vi "Periodic Tasks.vi"(8 "error in":errorcluster) -> ()   [LabVIEW 2014]
doc: "This VI runs in parallel to other tasks. It can contain as many user-defined periodic loops as you need. These can carry out PID or other sorts of timed response."
uses:
  <vilib>/Rock Robotics/WPI/DriverStation/WPI_DriverStationRobotMode2.ctl
  <vilib>/Rock Robotics/WPI/Solenoid/WPI_SolenoidValue.ctl
  <vilib>/Rock Robotics/WPI/RobotDrive/WPI_RobotDriveGetSetRefNum.vi
  <vilib>/Rock Robotics/WPI/Joystick/WPI_JoystickGetSetRefNum.vi
  <vilib>/Rock Robotics/Network Tables/SD Read Boolean.vi
  Robot Global Data.vi
  <vilib>/Rock Robotics/Network Tables/SD Write Boolean.vi
  <vilib>/addons/control/pid/pid.llb/PID (DBL).vi
  <vilib>/Rock Robotics/Network Tables/SD Write Number.vi
  <vilib>/Rock Robotics/WPI/Compressor/WPI_CompressorGetSetRefNum.vi
  Moose Code/Auto_Conf.vi
  <vilib>/Rock Robotics/WPI/Solenoid/WPI_SolenoidSetEnum.vi
  <vilib>/Rock Robotics/WPI/Solenoid/Deprecated/WPI_SolenoidSetBool.vi
  <vilib>/addons/control/pid/NI_PID_pid.lvlib
panel:
  out "Boolean":bool
  in  "Kpd":dbl=0.015
  in  "AllowZero":bool
  in  "ElevatorReset":bool
  out "GoatDetectorPhotoeye":bool
  out "D Contribution":dbl
  in  "Kd":dbl=0.025
  out "BottomOvertravel":bool=TRUE
  out "TopOvertravel":bool=TRUE
  out "ElevatorCurrent":dbl
  out "Voltage":dbl
  out "CurrentSum":dbl
  out "Motor Control":dbl(graph)
  in  "IZone":dbl=20.0
  out "Current":dbl
  out "Target":dbl
  out "PIDPhotoeye":bool
  in  "Kp":dbl=0.027
  in  "Ki":dbl=0.002 step=0.0001
  out "Target vs. Actual":T1(graph)
  out "I Contribution":dbl
  out "P Contribution":dbl
  in  "Threshold":dbl=5.5
  out "In Position":bool
  out "EncoderLeft":dbl
  out "EncoderRight":dbl
  # "K's as of 4-16-2015\nKp=0.027\nKpd=0.015\nKi=0.002\nKd=0.025\nIZone=20\nThreshold=5.5"
  # "K Tune-torial: (copied from Mindstorms docs)\n      Set the values of Ki, Kd"
  # "K Tune-torial: (copied from email)\n      Find a P gain that gets you close to your target without overshooting.  \nBased on that P gain value calculate the error at which your P starts to\ndecrease below full throttle.  Make your I cap equal to this error.  Make your\ninitial I gain very small (less than .1 say .0001).  The idea is to accumulate a \nvalue that is manageable. The Talon I accumulates every 1 millisecond so it\nis very easy to calculate the amount of time to get to full throttle.  An I gain\nof .001 will get you full throttle in about 1 second (assuming error never\nchanges).\n      The goal of this strategy is to make I perceivable while still allowing\nP to be the dominating component.  In position servo, I is only needed\nwhen P is not enough to get you to your target.  Once your P output is\nless than full throttle, I will start to kick in.  At first there will be a noticeable\ngap in throttle.  Throttle will decrease proportional to the error and then\nslowly ramp back up until the target is reached, this is useful in observing\nthe effect of I.  Slowly increase I and adjust the I zone until the throttle is \nalmost seamless."
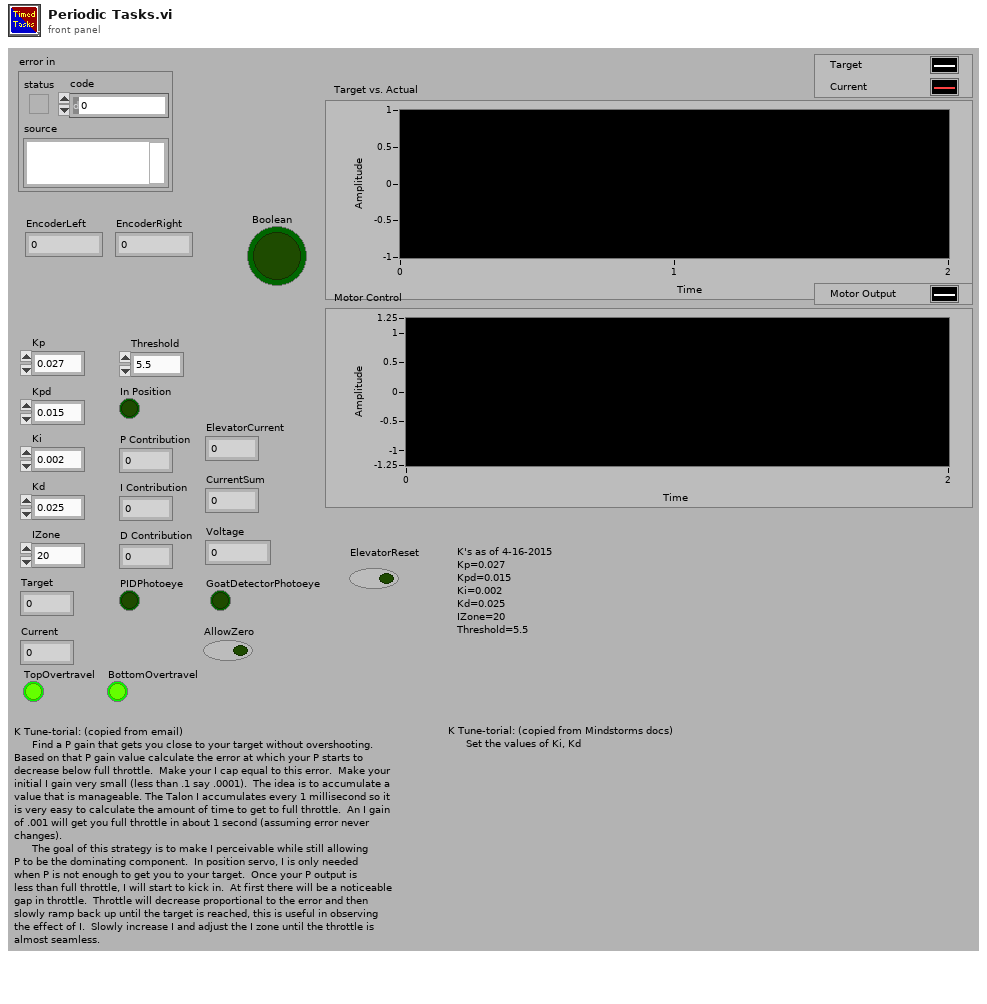
[diagram p1: front panel]
types:
  T1 = cluster{"[0]":dbl, "[1]":dbl, "[2]":dbl, "[3]":dbl, "[4]":dbl, "[5]":dbl, "[6]":dbl, "[7]":dbl, "[8]":dbl}
  T2 = enum16{"ResetForward", "ResetBack", "PIDControl", "ManualControl", "ZeroEncoderAndTarget", "AutoStack"}
  T3 = enum16{"Disabled", "Initialize", "CalcNewTarget", "Moving", "OpenArm", "CloseArm", "Reset"}
  T4 = typedef "WPI_EncoderDevRef.ctl" = cluster{"DevStatus":errorcluster, "EncoderIndex":T5, "CounterIndex":T6, "DistancePerCount":dbl, "Decoding Type":T7}
  T5 = typedef "FPGA_EncoderIdx.ctl" = enum8{"Enc 0", "Enc 1", "Enc 2", "Enc 3", "Enc 4", "Enc 5", "Enc 6", "Enc 7", "Invalid"}
  T6 = typedef "FPGA_CounterCtrSystemIndex.ctl" = enum8{"Ctr 0", "Ctr 1", "Ctr 2", "Ctr 3", "Ctr 4", "Ctr 5", "Ctr 6", "Ctr 7", "Invalid"}
  T7 = typedef "WPI_EncoderType.ctl" = enum16{"1x", "2x", "4x"}
  T8 = typedef "WPI_JoystickDevRef.ctl" = cluster{"Device":T9}
  T9 = typedef "WPI_JoystickDeviceEnum.ctl" = enum16{"USB 0", "USB 1", "USB 2", "USB 3", "USB 4", "USB 5"}
  T10 = typedef "WPI_SolenoidDevRef.ctl" = cluster{"DevStatus":errorcluster, "Pneumatics Control Module":u8, "Forward Solenoid Channel":T11, "Reverse Solenoid Channel":T11}
  T11 = typedef "WPI_SolenoidChannel.ctl" = enum8{"Solenoid 0", "Solenoid 1", "Solenoid 2", "Solenoid 3", "Solenoid 4", "Solenoid 5", "Solenoid 6", "Solenoid 7", "Invalid"}
  T12 = typedef "WPI_MotorControlDeviceRef.ctl" = cluster{"DeviceStatus":errorcluster, "Type":T13, "PWM":cluster{"Controller":T14, "PWM Channel":T15, "DeadBand":T16}, "CAN":cluster{"Device Number":u8, "Control Mode":T17, "Semaphore":T18, "Max Vout":dbl, "TalonSRX Control Mode":T19}, "Invert":bool, "TransformRef":T20, "InvTransformRef":T20}
  T13 = typedef "WPI_MotorControlType.ctl" = enum16{"PWM", "CAN", "CANTalonSRX"}
  T14 = typedef "FPGA_TypedefDigitalModule.ctl" = enum16{"Controller 1"}
  T15 = typedef "FPGA_DIOPWMChannel.ctl" = enum8{"PWM 0", "PWM 1", "PWM 2", "PWM 3", "PWM 4", "PWM 5", "PWM 6", "PWM 7", "PWM 8", "PWM 9", "PWM MXP 0", "PWM MXP 1", "PWM MXP 2", "PWM MXP 3", "PWM MXP 4", "PWM MXP 5", "PWM MXP 6", "PWM MXP 7", "PWM MXP 8", "PWM MXP 9", "Invalid"}
  T16 = typedef "WPI_PWMDeadband.ctl" = cluster{"Name":string, "maxPositivePwm":i32, "minPositivePwm":i32, "centerPwm":i32, "maxNegativePwm":i32, "minNegativePwm":i32, "angularRange":u16}
  T17 = typedef "WPI_CANJaguar_ControlMode.ctl" = enum8{"Percent VBus", "Current", "Speed", "Position", "Voltage"}
  T18 = typedef "Semaphore RefNum" = refnum<k1>
  T19 = typedef "WPI_CANTalonSRX_APIControlMode.ctl" = enum8{"Percent VBus", "Speed", "Position", "Slave", "Unchanged / Invalid"}
  T20 = typedef "WPI_PWMTransform_ConPane.ctl" = refnum<vi>
  T21 = typedef "WPI_RobotDriveDevRef.ctl" = cluster{"DevStatus":errorcluster, "Motors[]":T12[], "Square Inputs":bool, "Max Output":dbl}
  T22 = typedef "WPI_DigitalInputDevRef.ctl" = cluster{"DevStatus":errorcluster, "DIO Channel":T23, "Controller":T14}
  T23 = typedef "FPGA_DIOChannel.ctl" = enum8{"DIO 0", "DIO 1", "DIO 2", "DIO 3", "DIO 4", "DIO 5", "DIO 6", "DIO 7", "DIO 8", "DIO 9", "DIO MXP 0", "DIO MXP 1", "DIO MXP 2", "DIO MXP 3", "DIO MXP 4", "DIO MXP 5", "DIO MXP 6", "DIO MXP 7", "DIO MXP 8", "DIO MXP 9", "DIO MXP 10", "DIO MXP 11", "DIO MXP 12", "DIO MXP 13", "DIO MXP 14", "DIO MXP 15", "Invalid"}
  T24 = typedef "WPI_CompressorDevRef.ctl" = cluster{"DevStatus":errorcluster, "Pneumatics Control Module":u8}
  T25 = typedef "WPI_DriverStationRobotMode2.ctl" = enum16{"Autonomous Disabled", "Autonomous Enabled", "Teleop Disabled", "Teleop Enabled", "Disconnected", "Finish", "Test Disabled", "Test Enabled", "Emergency Stopped"}
  T26 = typedef "WPI_GyroDevRef.ctl" = cluster{"DevStatus":errorcluster, "Analog Module":T27, "Analog Channel":T28, "Offset":dbl, "Gain (VoltsPerDegree/Second)":dbl}
  T27 = typedef "FPGA_TypedefAnalogModule.ctl" = enum16{"Controller 1"}
  T28 = typedef "FPGA_AIChannel.ctl" = enum8{"AI 0", "AI 1", "AI 2", "AI 3", "AI MXP 0", "AI MXP 1", "AI MXP 2", "AI MXP 3", "Invalid"}
  T29 = typedef "WPI_SolenoidValue.ctl" = enum16{"Off", "On", "Forward", "Reverse"}
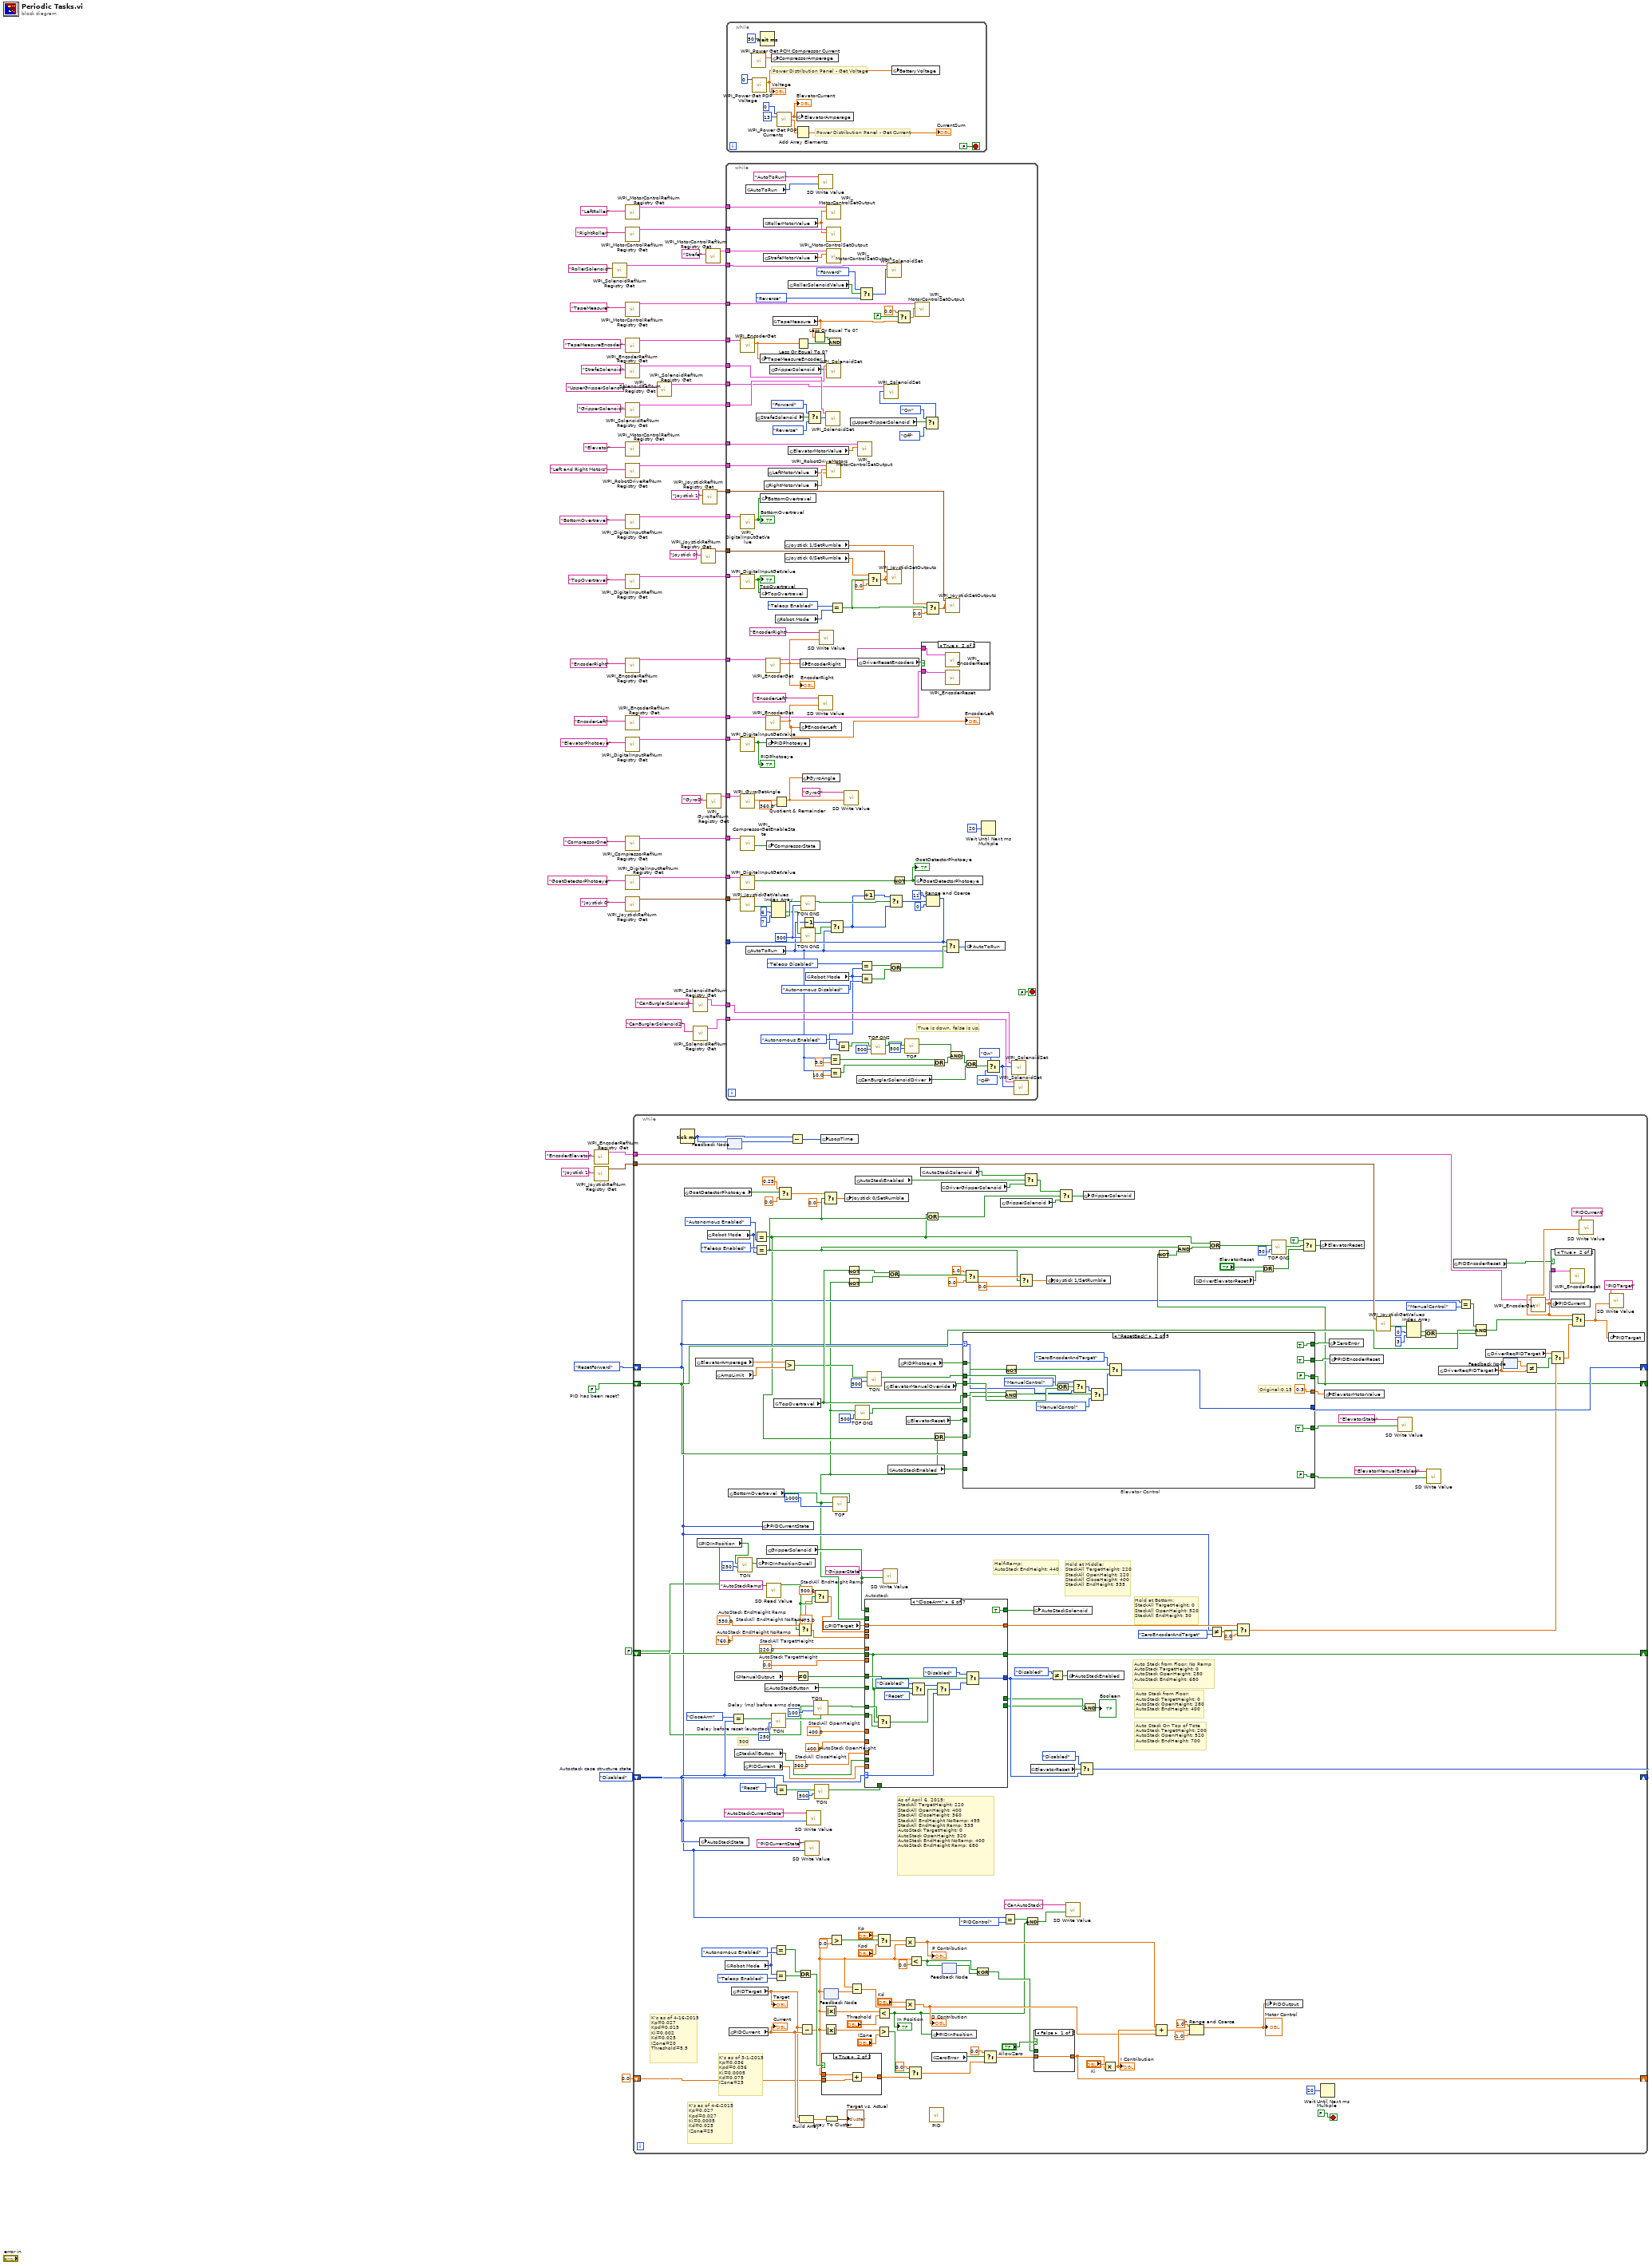
[diagram p0: block diagram]
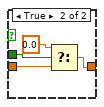
[diagram p4: hidden frame]
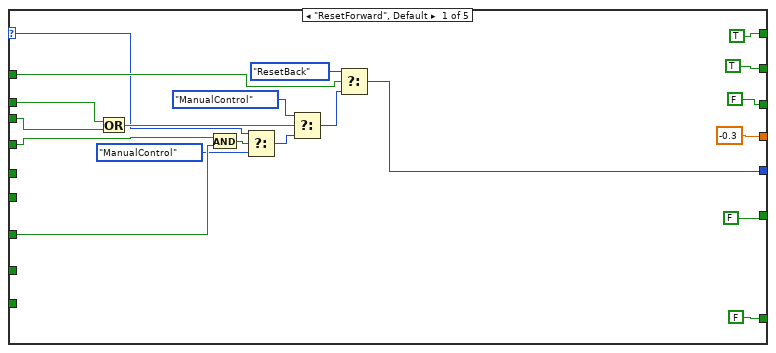
[diagram p5: hidden frame]
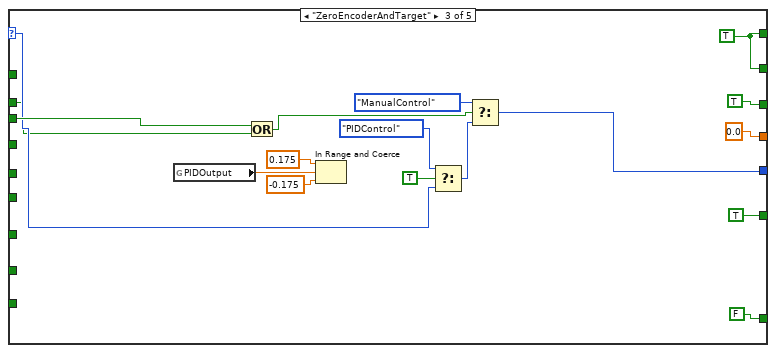
[diagram p6: hidden frame]
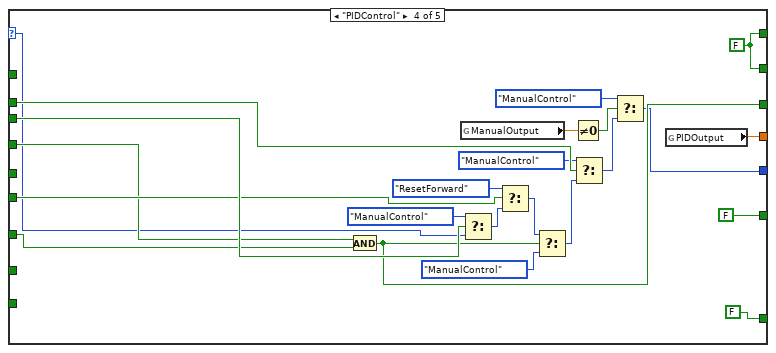
[diagram p7: hidden frame]
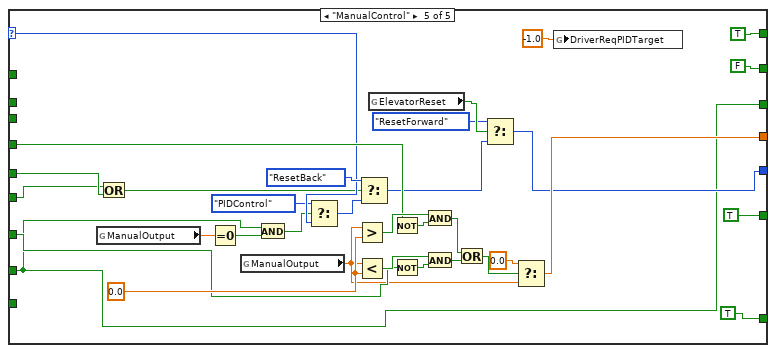
[diagram p8: hidden frame]
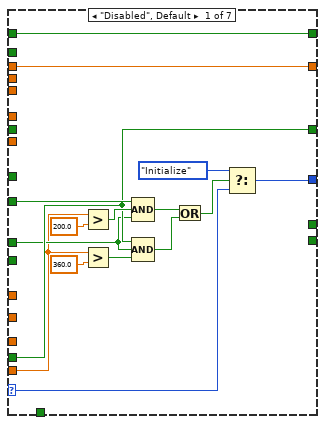
[diagram p9: hidden frame]
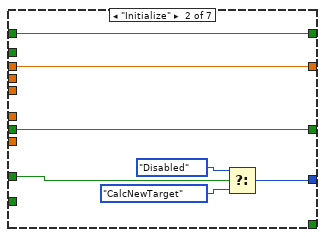
[diagram p10: hidden frame]
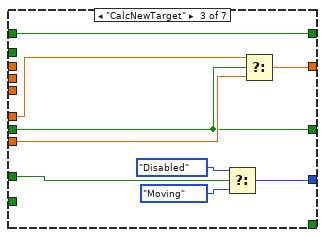
[diagram p11: hidden frame]
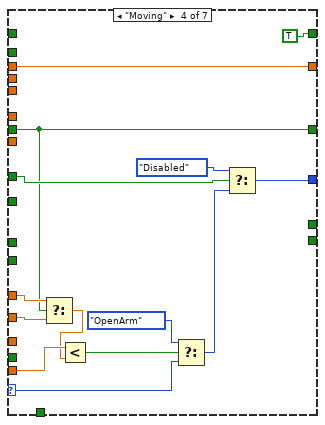
[diagram p12: hidden frame]
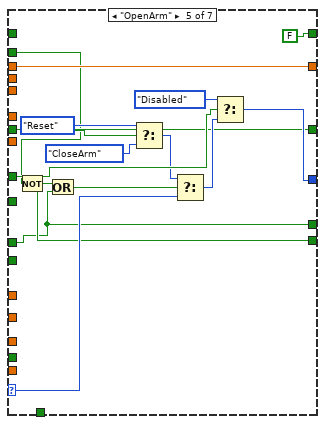
[diagram p13: hidden frame]
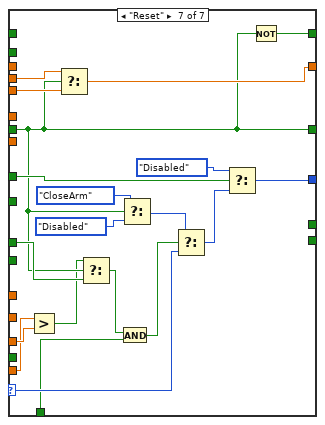
[diagram p14: hidden frame]
diagram:
  w28 = FALSE  # PID has been reset?
  w31 = T3."Disabled"  # Autostack case structure state
  n1 = call <vilib>:"WPI_EncoderRefNum Registry Get.vi"("refnum name"="EncoderElevator") -> ("EncoderDevRef"=w17:T4)  [unwired: 9 in, 1 out]
  n2 = call <vilib>:"WPI_JoystickRefNum Registry Get.vi"("refnum name"="Joystick 1") -> ("JoystickDevRef"=w15:T8)  [unwired: 9 in, 1 out]
  n3 = call <vilib>:"WPI_SolenoidRefNum Registry Get.vi"("refnum name"="RollerSolenoid") -> ("SolenoidDevRef"=w18:T10)  [unwired: 9 in, 1 out]
  n4 = call <vilib>:"WPI_MotorControlRefNum Registry Get.vi"("refnum name"="LeftRoller") -> ("MotorControlDevRef"=w21:T12)  [unwired: 9 in, 1 out]
  n5 = call <vilib>:"WPI_MotorControlRefNum Registry Get.vi"("refnum name"="RightRoller") -> ("MotorControlDevRef"=w20:T12)  [unwired: 9 in, 1 out]
  n6 = call <vilib>:"WPI_MotorControlRefNum Registry Get.vi"("refnum name"="TapeMeasure") -> ("MotorControlDevRef"=w12:T12)  [unwired: 9 in, 1 out]
  n7 = call <vilib>:"WPI_EncoderRefNum Registry Get.vi"("refnum name"="TapeMeasureEncoder") -> ("EncoderDevRef"=w9:T4)  [unwired: 9 in, 1 out]
  n8 = call <vilib>:"WPI_SolenoidRefNum Registry Get.vi"("refnum name"="StrafeSolenoid") -> ("SolenoidDevRef"=w24:T10)  [unwired: 9 in, 1 out]
  n9 = call <vilib>:"WPI_SolenoidRefNum Registry Get.vi"("refnum name"="GripperSolenoid") -> ("SolenoidDevRef"=w6:T10)  [unwired: 9 in, 1 out]
  n10 = call <vilib>:"WPI_MotorControlRefNum Registry Get.vi"("refnum name"="Elevator") -> ("MotorControlDevRef"=w5:T12)  [unwired: 9 in, 1 out]
  n11 = call <vilib>:"WPI_RobotDriveRefNum Registry Get.vi"("refnum name"="Left and Right Motors") -> ("RobotDriveDevRef"=w57:T21)  [unwired: 9 in, 1 out]
  n12 = call <vilib>:"WPI_DigitalInputRefNum Registry Get.vi"("refnum name"="BottomOvertravel") -> ("DigitalInputDevRef"=w39:T22)  [unwired: 9 in, 1 out]
  n13 = call <vilib>:"WPI_DigitalInputRefNum Registry Get.vi"("refnum name"="TopOvertravel") -> ("DigitalInputDevRef"=w41:T22)  [unwired: 9 in, 1 out]
  n14 = call <vilib>:"WPI_EncoderRefNum Registry Get.vi"("refnum name"="EncoderRight") -> ("EncoderDevRef"=w46:T4)  [unwired: 9 in, 1 out]
  n15 = call <vilib>:"WPI_EncoderRefNum Registry Get.vi"("refnum name"="EncoderLeft") -> ("EncoderDevRef"=w48:T4)  [unwired: 9 in, 1 out]
  n16 = call <vilib>:"WPI_DigitalInputRefNum Registry Get.vi"("refnum name"="ElevatorPhotoeye") -> ("DigitalInputDevRef"=w51:T22)  [unwired: 9 in, 1 out]
  n17 = call <vilib>:"WPI_CompressorRefNum Registry Get.vi"("refnum name"="CompressorOne") -> ("CompressorDevRef"=w13:T24)  [unwired: 9 in, 1 out]
  n18 = call <vilib>:"WPI_DigitalInputRefNum Registry Get.vi"("refnum name"="GoatDetectorPhotoeye") -> ("DigitalInputDevRef"=w32:T22)  [unwired: 9 in, 1 out]
  n19 = call <vilib>:"WPI_JoystickRefNum Registry Get.vi"("refnum name"="Joystick 0") -> ("JoystickDevRef"=w26:T8)  [unwired: 9 in, 1 out]
  n20 = while {
    shift-right: [w164] -> _
    shift-left: 0.0 -> [w103]
    shift-right: [w154] -> _
    shift-left: w31 -> [w85]
    shift-right: [w227] -> _
    shift-left: FALSE -> [w228]
    shift-right: [w189] -> _
    shift-left: T2."ResetForward" -> [w66]
    shift-right: [w97] -> _
    shift-left: w28 -> [w138]
    tunnel: w17 -> [w72]
    tunnel: w15 -> [w127]
    stop <- FALSE stop-if-true
    w68 = 475.0  # StackAll EndHeight NoRamp
    w70 = 500.0  # StackAll EndHeight Ramp
    w73 = 760.0  # AutoStack EndHeight NoRamp
    w82 = 360.0  # StackAll CloseHeight
    w91 = 400.0  # StackAll OpenHeight
    w90 = 400.0  # AutoStack OpenHeight
    w92 = 220.0  # StackAll TargetHeight
    w74 = 530.0  # AutoStack EndHeight Ramp
    w141 = 0.0  # AutoStack TargetHeight
    w148 = u32 250  # Delay before reset (autostack)
    w156 = u32 100  # Delay (ms) before arms close
    # "K's as of 4-16-2015\nKp=0.027\nKpd=0.015\nKi=0.002\nKd=0.025\nIZone=20\nThreshold=5.5"
    # "500"
    # "As of April 6, 2015:\nStackAll TargetHeight: 220\nStackAll OpenHeight: 400\nStackAll CloseHeight: 360\nStackAll EndHeight NoRamp: 495 \nStackAll EndHeight Ramp: 535\nAutoStack TargetHeight: 0\nAutoStack OpenHeight: 320\nAutoStack EndHeight NoRamp: 400\nAutoStack EndHeight Ramp: 680"
    # "K's as of 4-6-2015\nKp=0.027\nKpd=0.027\nKi=0.0005\nKd=0.025\nIZone=25"
    # "Auto Stack from Floor: No Ramp\nAutoStack TargetHeight: 0\nAutoStack OpenHeight: 280\nAutoStack EndHeight: 680"
    # "Half-Ramp:\nAutoStack EndHeight: 440"
    # "Hold at Bottom:\nStackAll TargetHeight: 0\nStackAll OpenHeight: 520\nStackAll EndHeight: 30"
    # "Auto Stack On Top of Tote\nAutoStack TargetHeight: 200\nAutoStack OpenHeight: 520\nAutoStack EndHeight: 700"
    # "Auto Stack from Floor:\nAutoStack TargetHeight: 0\nAutoStack OpenHeight: 280\nAutoStack EndHeight: 400"
    # "Hold at Middle:\nStackAll TargetHeight: 220\nStackAll OpenHeight: 220\nStackAll CloseHeight: 400\nStackAll EndHeight: 535"
    # "K's as of 3-1-2015\nKp=0.036\nKpd=0.036\nKi=0.0005\nKd=0.075\nIZone=25"
    n21 = Tick Count (ms)() -> (millisecond timer value=w173:u32)
    n22 = global read "Robot Global Data.vi" "GoatDetectorPhotoeye"() -> (w222:bool)
    n23 = global read "Robot Global Data.vi" "ElevatorAmperage"() -> (w200:dbl)
    n24 = global read "Robot Global Data.vi" "PIDInPosition"() -> (w63:bool)
    n25 = global write "Robot Global Data.vi" "AutoStackState"(w85) -> ()
    n26 = global read "Robot Global Data.vi" "Robot Mode"() -> (w98:T25)
    n27 = global read "Robot Global Data.vi" "AmpLimit"() -> (w201:dbl)
    n28 = global read "Robot Global Data.vi" "Robot Mode"() -> (w107:T25)
    n29 = feedback-in #1(w173) -> ()
    n30 = feedback #1() -> (w172:u32)  [unwired: 1 in]
    n31 = global read "Robot Global Data.vi" "BottomOvertravel"() -> (w62:bool)
    n32 = global read "Robot Global Data.vi" "PIDCurrent"() -> (w241:dbl)
    "Current" <- w241
    n33 = Equal?(x=T3."CloseArm" ("t"), y=w85) -> (x = y?=w149:bool)
    n34 = global read "Robot Global Data.vi" "PIDTarget"() -> (w237:dbl)
    "Target" <- w237
    n35 = global read "Robot Global Data.vi" "ManualOutput"() -> (w140:dbl)
    n36 = global read "Robot Global Data.vi" "StackAllButton"() -> (w83:bool)
    n37 = call "TON.vi"("Delay (ms)"=u32 250, "Input"=w63) -> ("Output"=w134:bool)  [unwired: 9 in]
    n38 = global read "Robot Global Data.vi" "PIDCurrent"() -> (w84:dbl)
    n39 = Equal?(x=w98, y=WPI_DriverStationRobotMode2."Autonomous Enabled") -> (x = y?=w113:bool)
    n40 = Equal?(x=WPI_DriverStationRobotMode2."Teleop Enabled" ("y"), y=w98) -> (x = y?=w115:bool)
    n41 = global write "Robot Global Data.vi" "PIDInPositionDwell"(w134) -> ()
    n42 = global write "Robot Global Data.vi" "PIDCurrentState"(w66) -> ()
    n43 = global read "Robot Global Data.vi" "AutoStackButton"() -> (w67:bool)
    n44 = global read "Robot Global Data.vi" "GripperSolenoid"() -> (w123:bool)
    n45 = call-poly <vilib>:"SD Read Value.vi"("Name"="AutoStackRamp") -> ("Boolean"=w71:bool)  [unwired: 8 in, 2 out]
    n46 = call "TON.vi"("Delay (ms)"=w148, "Input"=w149) -> ("Output"=w151:bool)  [unwired: 9 in]
    n47 = global read "Robot Global Data.vi" "TopOvertravel"() -> (w219:bool)
    n48 = Equal?(x=w107, y=WPI_DriverStationRobotMode2."Autonomous Enabled") -> (x = y?=w111:bool)
    n49 = Equal?(x=w107, y=WPI_DriverStationRobotMode2."Teleop Enabled") -> (x = y?=w110:bool)
    n50 = Equal?(x=T3."Reset" ("t"), y=w85) -> (x = y?=w88:bool)
    n51 = Select(t=0.25, s=w222, f=0.0) -> (s? t:f=w220:dbl)
    n52 = Greater?(x=w200, y=w201) -> (0:w202:bool)
    n53 = Subtract(x=w173, y=w172) -> (x-y=w171:u32)
    n54 = Not Equal To 0?(x=w140) -> (x != 0?=w139:bool)
    n55 = Select(t=w74, s=w71, f=w73) -> (s? t:f=w76:dbl)
    n56 = Or(x=w111, y=w110) -> (x .or. y?=w106:bool)
    n57 = Build Array(w237, w241) -> (w245:dbl[])
    n58 = Subtract(x=w237, y=w241) -> (x-y=w104:dbl)
    n59 = call-poly <vilib>:"SD Write Value.vi"("Numeric"=w66, "Name"="PIDCurrentState") -> ()  [unwired: 8 in, 2 out]
    n60 = call-poly <vilib>:"SD Write Value.vi"("Numeric"=w85, "Name"="AutoStackCurrentState") -> ()  [unwired: 8 in, 2 out]
    n61 = call "TON.vi"("Delay (ms)"=w156, "Input"=w63) -> ("Output"=w119:bool)  [unwired: 9 in]
    n62 = Select(t=w70, s=w71, f=w68) -> (s? t:f=w69:dbl)
    n63 = call "TON.vi"("Delay (ms)"=u32 500, "Input"=w88) -> ("Output"=w86:bool)  [unwired: 9 in]
    n64 = global write "Robot Global Data.vi" "LoopTime"(w171) -> ()
    n65 = case shown="True" w106 {
      tunnel: [w252 w255] -> w105
      tunnel: w104 -> [_ w254]
      tunnel: w103 -> [w252 w253]
      frame False {
      }
      frame True {
        n66 = Add(x=w254, y=w253) -> (x+y=w255:dbl)
      }
    }
    n67 = Select(t=w220, s=w115, f=0.0) -> (s? t:f=w205:dbl)
    n68 = global read "Robot Global Data.vi" "PIDTarget"() -> (w229:dbl)
    n69 = Absolute Value(x=w104) -> (abs(x)=w243:dbl)
    n70 = Absolute Value(x=w104) -> (abs(x)=w240:dbl)
    n71 = feedback-in #2(w104) -> ()
    n72 = feedback #2() -> (w236:dbl)  [unwired: 1 in]
    n73 = Array To Cluster(array=w245) -> (cluster=→"Target vs. Actual":T1)
    n74 = Greater?(x=w104, y=0.0) -> (0:w146:bool)
    n75 = call "TOF.vi"("Delay (ms)"=u32 1000, "Input"=w62) -> ("Output"=w65:bool)  [unwired: 9 in]
    n76 = global write "Robot Global Data.vi" "Joystick 0/SetRumble"(w205) -> ()
    n77 = Not(x=w219) -> (.not. x?=w217:bool)
    n78 = Not(x=w65) -> (.not. x?=w218:bool)
    n79 = Subtract(x=w104, y=w236) -> (x-y=w234:dbl)
    n80 = global read "Robot Global Data.vi" "AutoStackEnabled"() -> (w102:bool)
    n81 = call "TOF ONS.vi"("Delay (ms)"=u32 500, "Input"=w65) -> ("Output"=w136:bool)  [unwired: 9 in]
    n82 = case "Autostack" shown="\"CloseArm\"" w85 {
      selector: w85 -> [w391 _ _ w420 w434 w449 w470]
      tunnel: w141 -> [_ _ w405 _ _ _ _]
      tunnel: w67 -> [w382 _ _ _ _ _ _]
      tunnel: w229 -> [w376 w398 _ w417 w435 w450 _]
      tunnel: [w376 w398 w407 w417 w435 w450 w469] -> w186
      tunnel: w83 -> [w381 _ _ _ _ _ _]
      tunnel: [w381 w397 w400 w409 w429 w437 w455] -> w227
      tunnel: w228 -> [_ w397 w400 w409 w429 w437 w455]
      tunnel: [w387 w396 w406 TRUE FALSE ("Solenoid") TRUE ("Solenoid") w463] -> w230
      tunnel: w123 -> [w387 w396 w406 _ _ _ _]
      tunnel: [w389 w393 w402 w416 w433 w447 w466] -> w155
      tunnel: w119 -> [w379 _ _ _ w422 w440 w456]
      tunnel: w84 -> [w377 _ _ w412 _ _ w452]
      tunnel: w151 -> [_ _ _ _ _ w439 _]
      tunnel: w69 -> [_ _ _ _ _ _ w468]
      tunnel: w139 -> [_ w392 w401 w414 w430 w441 w459]
      tunnel: w76 -> [_ _ _ _ _ _ w464]
      tunnel: w92 -> [_ _ w399 _ _ _ _]
      tunnel: w91 -> [_ _ _ w411 _ _ _]
      tunnel: w90 -> [_ _ _ w410 _ _ _]
      tunnel: w86 -> [_ _ _ _ _ _ w457]
      tunnel: w82 -> [_ _ _ _ _ _ w453]
      tunnel: w62 -> [_ _ _ _ w424 _ _]
      tunnel: [_ _ _ _ w423 _ _] -> w60
      tunnel: [_ _ _ _ w422 _ _] -> w59
      frame "Disabled", Default {
        n83 = Greater?(x=w377, y=200.0) -> (0:w388:bool)
        n84 = Greater?(x=w377, y=360.0) -> (0:w378:bool)
        n85 = Compound Arithmetic op=AND(w382, w388, w379) -> (w385:bool)
        n86 = Compound Arithmetic op=AND(w381, w379, w378) -> (w383:bool)
        n87 = Or(x=w385, y=w383) -> (x .or. y?=w384:bool)
        n88 = Select(t=T3."Initialize", s=w384, f=w391) -> (s? t:f=w389:T3)
      }
      frame "Initialize" {
        n89 = Select(t=T3."Disabled", s=w392, f=T3."CalcNewTarget") -> (s? t:f=w393:T3)
      }
      frame "CalcNewTarget" {
        n90 = Select(t=T3."Disabled", s=w401, f=T3."Moving") -> (s? t:f=w402:T3)
        n91 = Select(t=w399, s=w400, f=w405) -> (s? t:f=w407:dbl)
      }
      frame "Moving" {
        n92 = Select(t=w411, s=w409, f=w410) -> (s? t:f=w408:dbl)
        n93 = Less?(x=w412, y=w408) -> (x < y?=w421:bool)
        n94 = Select(t=T3."OpenArm", s=w421, f=w420) -> (s? t:f=w415:T3)
        n95 = Select(t=T3."Disabled", s=w414, f=w415) -> (s? t:f=w416:T3)
      }
      frame "OpenArm" {
        n96 = Not(x=w424) -> (.not. x?=w423:bool)
        n97 = Or(x=w423, y=w422) -> (x .or. y?=w425:bool)
        n98 = Select(t=T3."Reset", s=w429, f=T3."CloseArm" ("t")) -> (s? t:f=w426:T3)
        n99 = Select(t=w426, s=w425, f=w434) -> (s? t:f=w432:T3)
        n100 = Select(t=T3."Disabled", s=w430, f=w432) -> (s? t:f=w433:T3)
      }
      frame "CloseArm" {
        n101 = Select(t=w440, s=w437, f=w439) -> (s? t:f=w438:bool)
        n102 = Select(t=T3."Disabled", s=w437, f=T3."Reset" ("t")) -> (s? t:f=w442:T3)
        n103 = Select(t=w442, s=w438, f=w449) -> (s? t:f=w446:T3)
        n104 = Select(t=T3."Disabled", s=w441, f=w446) -> (s? t:f=w447:T3)
      }
      frame "Reset" {
        n105 = Greater?(x=w452, y=w453) -> (0:w451:bool)
        n106 = Select(t=w468, s=w455, f=w464) -> (s? t:f=w469:dbl)
        n107 = Select(t=w451, s=w455, f=w456) -> (s? t:f=w454:bool)
        n108 = And(x=w454, y=w457) -> (x .and. y?=w458:bool)
        n109 = Select(t=T3."CloseArm", s=w455, f=T3."Disabled" ("t")) -> (s? t:f=w460:T3)
        n110 = Select(t=w460, s=w458, f=w470) -> (s? t:f=w465:T3)
        n111 = Select(t=T3."Disabled", s=w459, f=w465) -> (s? t:f=w466:T3)
        n112 = Not(x=w455) -> (.not. x?=w463:bool)
      }
    }
    n113 = call "TON.vi"("Delay (ms)"=u32 500, "Input"=w202) -> ("Output"=w203:bool)  [unwired: 9 in]
    n114 = Greater?(x=w240, y="IZone") -> (0:w181:bool)
    n115 = Select(t="Kp", s=w146, f="Kpd") -> (s? t:f=w145:dbl)
    n116 = Less?(x=w243, y="Threshold") -> (x < y?=w94:bool)
    "In Position" <- w94
    n117 = call-poly <vilib>:"SD Write Value.vi"("Boolean"=w123, "Name"="GripperState") -> ()  [unwired: 8 in, 2 out]
    n118 = global read "Robot Global Data.vi" "ElevatorManualOverride"() -> (w194:bool)
    n119 = Or(x=w217, y=w218) -> (x .or. y?=w215:bool)
    n120 = global read "Robot Global Data.vi" "AutoStackEnabled"() -> (w101:bool)
    n121 = global read "Robot Global Data.vi" "PIDPhotoeye"() -> (w193:bool)
    n122 = Multiply(x=w145, y=w104) -> (x*y=w182:dbl)
    "P Contribution" <- w182
    n123 = Multiply(x="Kd", y=w234) -> (x*y=w233:dbl)
    "D Contribution" <- w233
    n124 = global read "Robot Global Data.vi" "ElevatorReset"() -> (w195:bool)
    n125 = Select(t=0.0, s=w181, f=w105) -> (s? t:f=w158:dbl)
    n126 = Less?(x=w104, y=0.0) -> (x < y?=w167:bool)
    n127 = global read "Robot Global Data.vi" "AutoStackSolenoid"() -> (w209:bool)
    n128 = Or(x=w113, y=w115) -> (x .or. y?=w211:bool)
    n129 = call-poly <vilib>:"PID.vi"() -> ()  [unwired: 10 in, 2 out]
    n130 = global write "Robot Global Data.vi" "PIDInPosition"(w94) -> ()
    n131 = global read "Robot Global Data.vi" "ZeroError"() -> (w160:bool)
    n132 = Or(x=w65, y=w113) -> (x .or. y?=w120:bool)
    n133 = global read "Robot Global Data.vi" "DriverGripperSolenoid"() -> (w208:bool)
    n134 = feedback-in #3(w167) -> ()
    n135 = feedback #3() -> (w166:bool)  [unwired: 1 in]
    n136 = case "Elevator Control" shown="\"ResetBack\"" w66 {
      selector: w66 -> [w263 w284 w314 w324 w355]
      tunnel: [-0.3 0.3 0.0 ("ManualOutput") w323 w374] -> w192
      tunnel: [w265 w285 w319 w320 w345] -> w189
      tunnel: w193 -> [w280 w301 _ _ _]
      tunnel: w194 -> [w267 w299 w318 w342 _]
      tunnel: w195 -> [_ _ _ w341 w351]
      tunnel: [TRUE ("PIDEncoderReset") TRUE ("PIDEncoderReset") w310 w339 FALSE ("PIDEncoderReset")] -> w199
      tunnel: [TRUE ("PIDEncoderReset") TRUE ("PIDEncoderReset") w310 w339 TRUE ("PIDEncoderReset")] -> w117
      tunnel: w219 -> [w277 w295 _ w336 w372]
      tunnel: w120 -> [w276 w294 _ w335 w366]
      tunnel: w203 -> [w269 w291 w308 w334 _]
      tunnel: [FALSE ("PIDEncoderReset") FALSE ("PIDEncoderReset") FALSE ("PIDEncoderReset") FALSE ("PIDEncoderReset") TRUE ("PIDEncoderReset")] -> w179
      tunnel: w101 -> [_ _ _ _ _]
      tunnel: w138 -> [_ _ _ _ w343]
      tunnel: [FALSE FALSE TRUE w321 w343] -> w97
      tunnel: w136 -> [_ _ _ _ w352]
      tunnel: [FALSE ("PIDEncoderReset") TRUE ("PIDEncoderReset") TRUE ("PIDEncoderReset") FALSE ("PIDEncoderReset") TRUE ("PIDEncoderReset")] -> w121
      frame "ResetForward", Default {
        n137 = Or(x=w269, y=w267) -> (x .or. y?=w268:bool)
        n138 = And(x=w277, y=w276) -> (x .and. y?=w278:bool)
        n139 = Select(t=w263, s=w278, f=T2."ManualControl") -> (s? t:f=w273:T2)
        n140 = Select(t=T2."ManualControl", s=w268, f=w273) -> (s? t:f=w264:T2)
        n141 = Select(t=T2."ResetBack", s=w280, f=w264) -> (s? t:f=w265:T2)
      }
      frame "ResetBack" {
        # "Original:0.15"
        n142 = Not(x=w301) -> (.not. x?=w300:bool)
        n143 = And(x=w295, y=w294) -> (x .and. y?=w297:bool)
        n144 = Or(x=w291, y=w299) -> (x .or. y?=w292:bool)
        n145 = Select(t=T2."ManualControl", s=w292, f=w284) -> (s? t:f=w296:T2)
        n146 = Select(t=w296, s=w297, f=T2."ManualControl") -> (s? t:f=w283:T2)
        n147 = Select(t=T2."ZeroEncoderAndTarget", s=w300, f=w283) -> (s? t:f=w285:T2)
      }
      frame "ZeroEncoderAndTarget" {
        w310 = TRUE ("PIDEncoderReset")
        n148 = global read "Robot Global Data.vi" "PIDOutput"() -> (w313:dbl)
        n149 = Or(x=w318, y=w308) -> (x .or. y?=w309:bool)
        n150 = In Range and Coerce(upper limit=0.175, x=w313, lower limit=-0.175) -> ()  [unwired: 2 out]
        n151 = Select(t=T2."PIDControl", s=TRUE, f=w314) -> (s? t:f=w316:T2)
        n152 = Select(t=T2."ManualControl", s=w309, f=w316) -> (s? t:f=w319:T2)
      }
      frame "PIDControl" {
        w339 = FALSE ("PIDEncoderReset")
        n153 = And(x=w336, y=w335) -> (x .and. y?=w321:bool)
        n154 = global read "Robot Global Data.vi" "ManualOutput"() -> (w326:dbl)
        n155 = Select(t=T2."ManualControl", s=w342, f=w324) -> (s? t:f=w340:T2)
        n156 = Select(t=T2."ResetForward", s=w341, f=w340) -> (s? t:f=w337:T2)
        n157 = Select(t=w337, s=w321, f=T2."ManualControl") -> (s? t:f=w338:T2)
        n158 = Not Equal To 0?(x=w326) -> (x != 0?=w325:bool)
        n159 = Select(t=T2."ManualControl", s=w334, f=w338) -> (s? t:f=w328:T2)
        n160 = Select(t=T2."ManualControl", s=w325, f=w328) -> (s? t:f=w320:T2)
        n161 = global read "Robot Global Data.vi" "PIDOutput"() -> (w323:dbl)
      }
      frame "ManualControl" {
        w368 = 0.0 ("y")
        n162 = global read "Robot Global Data.vi" "ManualOutput"() -> (w358:dbl)
        n163 = Or(x=w351, y=w352) -> (x .or. y?=w350:bool)
        n164 = Equal To 0?(x=w358) -> (x = 0?=w357:bool)
        n165 = global read "Robot Global Data.vi" "ManualOutput"() -> (w364:dbl)
        n166 = And(x=w343, y=w357) -> (x .and. y?=w353:bool)
        n167 = Select(t=T2."PIDControl", s=w353, f=w355) -> (s? t:f=w356:T2)
        n168 = Greater?(x=w364, y=w368) -> (0:w373:bool)
        n169 = Less?(x=w364, y=w368) -> (x < y?=w367:bool)
        n170 = Select(t=T2."ResetBack", s=w350, f=w356) -> (s? t:f=w346:T2)
        n171 = global read "Robot Global Data.vi" "ElevatorReset"() -> (w347:bool)
        n172 = Not(x=w372) -> (.not. x?=w362:bool)
        n173 = Not(x=w366) -> (.not. x?=w363:bool)
        n174 = And(x=w373, y=w362) -> (x .and. y?=w370:bool)
        n175 = And(x=w367, y=w363) -> (x .and. y?=w365:bool)
        n176 = Or(x=w370, y=w365) -> (x .or. y?=w369:bool)
        n177 = Select(t=T2."ResetForward", s=w347, f=w346) -> (s? t:f=w345:T2)
        n178 = Select(t=0.0, s=w369, f=w364) -> (s? t:f=w374:dbl)
        n179 = global write "Robot Global Data.vi" "DriverReqPIDTarget"(-1.0 ("DriverReqPIDTarget")) -> ()
      }
    }
    n180 = Select(t=1.0, s=w215, f=0.0) -> (s? t:f=w214:dbl)
    n181 = Exclusive Or(1:w166, 2:w167) -> (0:w163:bool)
    n182 = Select(t=0.0, s=w160, f=w158) -> (s? t:f=w161:dbl)
    n183 = global read "Robot Global Data.vi" "GripperSolenoid"() -> (w212:bool)
    n184 = Equal?(x=w66, y=T2."PIDControl") -> (x = y?=w95:bool)
    n185 = Select(t=w214, s=w115, f=0.0) -> (s? t:f=w206:dbl)
    n186 = Select(t=w209, s=w102, f=w208) -> (s? t:f=w210:bool)
    n187 = And(x=w95, y=w94) -> (x .and. y?=w93:bool)
    n188 = global read "Robot Global Data.vi" "ElevatorReset"() -> (w153:bool)
    n189 = global write "Robot Global Data.vi" "AutoStackSolenoid"(w230) -> ()
    n190 = case shown="False" "AllowZero" {
      tunnel: [w257 w261] -> w164
      tunnel: w163 -> [_ w260]
      tunnel: w161 -> [w257 w259]
      frame False {
      }
      frame True {
        n191 = Select(t=0.0, s=w260, f=w259) -> (s? t:f=w261:dbl)
      }
    }
    n192 = global write "Robot Global Data.vi" "Joystick 1/SetRumble"(w206) -> ()
    n193 = Not Equal?(x=T3."Disabled", y=w155) -> (x != y?=w232:bool)
    n194 = Select(t=w210, s=w211, f=w212) -> (s? t:f=w142:bool)
    n195 = call-poly <vilib>:"SD Write Value.vi"("Boolean"=w93, "Name"="CanAutoStack") -> ()  [unwired: 8 in, 2 out]
    n196 = global write "Robot Global Data.vi" "AutoStackEnabled"(w232) -> ()
    n197 = Select(t=T3."Disabled", s=w153, f=w155) -> (s? t:f=w154:T3)
    n198 = global write "Robot Global Data.vi" "GripperSolenoid"(w142) -> ()
    n199 = And(x=w60, y=w59) -> (x .and. y?=→"Boolean":bool)
    n200 = Multiply(x="Ki", y=w164) -> (x*y=w250:dbl)
    "I Contribution" <- w250
    n201 = Not(x=w97) -> (.not. x?=w116:bool)
    n202 = Compound Arithmetic op=ADD(w182, w250, w233) -> (w246:dbl)
    n203 = And(x=w115, y=w116) -> (x .and. y?=w114:bool)
    n204 = In Range and Coerce(upper limit=1.0, x=w246, lower limit=-1.0) -> (coerced(x)=w238:dbl)  [unwired: 1 out]
    "Motor Control" <- w238
    n205 = global read "Robot Global Data.vi" "DriverElevatorReset"() -> (w224:bool)
    n206 = Or(x=w113, y=w114) -> (x .or. y?=w112:bool)
    n207 = Not Equal?(x=w66, y=T2."ZeroEncoderAndTarget") -> (x != y?=w188:bool)
    n208 = Select(t=w186, s=w188, f=0.0) -> (s? t:f=w175:dbl)
    n209 = Or(x="ElevatorReset", y=w224) -> (x .or. y?=w226:bool)
    n210 = global write "Robot Global Data.vi" "PIDOutput"(w238) -> ()
    n211 = call "TOF ONS.vi"("Delay (ms)"=u32 50, "Input"=w112) -> ("Output"=w196:bool)  [unwired: 9 in]
    n212 = Select(t=TRUE, s=w196, f=w226) -> (s? t:f=w198:bool)
    n213 = global write "Robot Global Data.vi" "ElevatorReset"(w198) -> ()
    n214 = Wait Until Next ms Multiple(millisecond multiple=u32 20) -> ()  [unwired: 1 out]
    n215 = global write "Robot Global Data.vi" "ElevatorMotorValue"(w192) -> ()
    n216 = global write "Robot Global Data.vi" "ZeroError"(w117) -> ()
    n217 = global write "Robot Global Data.vi" "PIDEncoderReset"(w199) -> ()
    n218 = call <vilib>:"WPI_JoystickGetValues.vi"("JoystickDevRef"=w127) -> ("Buttons"=w130:bool[])  [unwired: 6 in, 4 out]
    n219 = call-poly <vilib>:"SD Write Value.vi"("Boolean"=w121, "Name"="ElevatorState") -> ()  [unwired: 8 in, 2 out]
    n220 = Index Array(array=w130, index #1=0 ("index"), index #2=3 ("index")) -> (element #1=w126:bool, element #2=w125:bool)
    n221 = Or(x=w126, y=w125) -> (x .or. y?=w81:bool)
    n222 = call-poly <vilib>:"SD Write Value.vi"("Boolean"=w179, "Name"="ElevatorManualEnabled") -> ()  [unwired: 8 in, 2 out]
    n223 = global read "Robot Global Data.vi" "DriverReqPIDTarget"() -> (w170:dbl)
    n224 = global read "Robot Global Data.vi" "PIDEncoderReset"() -> (w58:bool)
    n225 = Equal?(x=w66, y=T2."ManualControl") -> (x = y?=w183:bool)
    n226 = Compound Arithmetic op=AND(w183, w138, w81) -> (w180:bool)
    n227 = global read "Robot Global Data.vi" "DriverReqPIDTarget"() -> (w176:dbl)
    n228 = feedback-in #4(w170) -> ()
    n229 = feedback #4() -> (w169:dbl)  [unwired: 1 in]
    n230 = Not Equal?(x=w169, y=w170) -> (x != y?=w177:bool)
    n231 = call <vilib>:"WPI_EncoderGet.vi"("EncoderDevRef"=w72) -> ("Distance"=w77:dbl, "EncoderDevRef"=w131:T4)  [unwired: 5 in, 4 out]
    n232 = Select(t=w176, s=w177, f=w175) -> (s? t:f=w174:dbl)
    n233 = case shown="True" w58 {
      tunnel: w131 -> [_ w256]
      frame False {
      }
      frame True {
        n234 = call <vilib>:"WPI_EncoderReset.vi"("EncoderDevRef"=w256) -> ()  [unwired: 9 in, 2 out]
      }
    }
    n235 = global write "Robot Global Data.vi" "PIDCurrent"(w77) -> ()
    n236 = Select(t=w77, s=w180, f=w174) -> (s? t:f=w80:dbl)
    n237 = call-poly <vilib>:"SD Write Value.vi"("Numeric"=w77, "Name"="PIDCurrent") -> ()  [unwired: 8 in, 2 out]
    n238 = global write "Robot Global Data.vi" "PIDTarget"(w80) -> ()
    n239 = call-poly <vilib>:"SD Write Value.vi"("Numeric"=w80, "Name"="PIDTarget") -> ()  [unwired: 8 in, 2 out]
  }
  n240 = call <vilib>:"WPI_SolenoidRefNum Registry Get.vi"("refnum name"="UpperGripperSolenoid") -> ("SolenoidDevRef"=w7:T10)  [unwired: 9 in, 1 out]
  n241 = call <vilib>:"WPI_SolenoidRefNum Registry Get.vi"("refnum name"="CanBurglarSolenoid") -> ("SolenoidDevRef"=w3:T10)  [unwired: 9 in, 1 out]
  n242 = call <vilib>:"WPI_SolenoidRefNum Registry Get.vi"("refnum name"="CanBurglarSolenoid2") -> ("SolenoidDevRef"=w1:T10)  [unwired: 9 in, 1 out]
  n243 = call <vilib>:"WPI_JoystickRefNum Registry Get.vi"("refnum name"="Joystick 0") -> ("JoystickDevRef"=w34:T8)  [unwired: 1 in, 9 out]
  n244 = call <vilib>:"WPI_JoystickRefNum Registry Get.vi"("refnum name"="Joystick 1") -> ("JoystickDevRef"=w35:T8)  [unwired: 1 in, 9 out]
  n245 = call <vilib>:"WPI_MotorControlRefNum Registry Get.vi"("refnum name"="Strafe") -> ("MotorControlDevRef"=w54:T12)  [unwired: 9 in, 1 out]
  n246 = call <vilib>:"WPI_GyroRefNum Registry Get.vi"("refnum name"="Gyro0") -> ("GyroDevRef"=w44:T26)  [unwired: 9 in, 1 out]
  n247 = while {
    tunnel: w57 -> [w589]
    tunnel: w54 -> [w588]
    tunnel: w5 -> [w583]
    tunnel: w51 -> [w582]
    tunnel: w48 -> [w581]
    tunnel: w46 -> [w580]
    tunnel: w44 -> [w578]
    tunnel: w41 -> [w575]
    tunnel: w39 -> [w574]
    tunnel: w6 -> [w573]
    tunnel: w35 -> [w537]
    tunnel: w34 -> [w530]
    tunnel: w32 -> [w569]
    tunnel: w26 -> [w545]
    tunnel: w24 -> [w544]
    tunnel: w21 -> [w528]
    tunnel: w20 -> [w527]
    tunnel: w18 -> [w526]
    tunnel: w13 -> [w520]
    tunnel: w12 -> [w518]
    tunnel: w9 -> [w516]
    tunnel: w7 -> [w502]
    tunnel: w3 -> [w497]
    tunnel: [w490] -> _
    tunnel: w1 -> [w486]
    stop <- FALSE stop-if-true
    w552 = u32 500 ("Delay (ms)")
    # "True is down, false is up."
    n248 = call <vilib>:"WPI_EncoderGet.vi"("EncoderDevRef"=w516) -> ("Distance"=w503:dbl)  [unwired: 5 in, 5 out]
    n249 = call <vilib>:"WPI_DigitalInputGetValue.vi"("DigitalInputDevRef"=w574) -> ("Value"=w571:bool)  [unwired: 8 in, 2 out]
    "BottomOvertravel" <- w571
    n250 = call <vilib>:"WPI_DigitalInputGetValue.vi"("DigitalInputDevRef"=w575) -> ("Value"=w572:bool)  [unwired: 8 in, 2 out]
    "TopOvertravel" <- w572
    n251 = call <vilib>:"WPI_DigitalInputGetValue.vi"("DigitalInputDevRef"=w582) -> ("Value"=w579:bool)  [unwired: 8 in, 2 out]
    "PIDPhotoeye" <- w579
    n252 = call <vilib>:"WPI_GyroGetAngle.vi"("GyroDevRef"=w578) -> ("Angle"=w577:dbl)  [unwired: 7 in, 3 out]
    n253 = call <vilib>:"WPI_CompressorGetEnableState.vi"("CompressorDevRef"=w520) -> ("Compressor Running"=w519:bool)  [unwired: 7 in, 3 out]
    n254 = call <vilib>:"WPI_DigitalInputGetValue.vi"("DigitalInputDevRef"=w569) -> ("Value"=w570:bool)  [unwired: 8 in, 2 out]
    n255 = call <vilib>:"WPI_JoystickGetValues.vi"("JoystickDevRef"=w545) -> ("Buttons"=w549:bool[])  [unwired: 6 in, 4 out]
    n256 = global read "Auto_Conf.vi" "AutoToRun"() -> (w557:u8)
    n257 = global read "Auto_Conf.vi" "AutoToRun"() -> (w473:u8)
    n258 = global read "Robot Global Data.vi" "StrafeSolenoid"() -> (w541:bool)
    n259 = global write "Robot Global Data.vi" "TapeMeasureEncoder"(w503) -> ()
    n260 = global write "Robot Global Data.vi" "BottomOvertravel"(w571) -> ()
    n261 = global write "Robot Global Data.vi" "TopOvertravel"(w572) -> ()
    n262 = global read "Robot Global Data.vi" "RollerMotorValue"() -> (w505:dbl)
    n263 = global read "Robot Global Data.vi" "StrafeMotorValue"() -> (w587:dbl)
    n264 = global read "Robot Global Data.vi" "RightMotorValue"() -> (w585:dbl)
    n265 = call <vilib>:"WPI_EncoderGet.vi"("EncoderDevRef"=w580) -> ("Distance"=w509:dbl, "EncoderDevRef"=w492:T4)  [unwired: 5 in, 4 out]
    "EncoderRight" <- w509
    n266 = call <vilib>:"WPI_EncoderGet.vi"("EncoderDevRef"=w581) -> ("Distance"=w507:dbl, "EncoderDevRef"=w491:T4)  [unwired: 5 in, 4 out]
    "EncoderLeft" <- w507
    n267 = global write "Robot Global Data.vi" "PIDPhotoeye"(w579) -> ()
    n268 = global write "Robot Global Data.vi" "CompressorState"(w519) -> ()
    n269 = global read "Robot Global Data.vi" "LeftMotorValue"() -> (w586:dbl)
    n270 = global read "Robot Global Data.vi" "GripperSolenoid"() -> (w543:bool)
    n271 = Index Array(array=w549, index #1=6 ("index"), index #2=7 ("index")) -> (element #1=w550:bool, element #2=w551:bool)
    n272 = global read "Robot Global Data.vi" "TapeMeasure"() -> (w511:dbl)
    n273 = Quotient & Remainder(x=w577, y=360.0) -> (x-y*floor(x/y)=w521:dbl)  [unwired: 1 out]
    n274 = global read "Robot Global Data.vi" "Robot Mode"() -> (w539:T25)
    n275 = global read "Robot Global Data.vi" "Joystick 1/SetRumble"() -> (w488:dbl)
    n276 = global read "Robot Global Data.vi" "Joystick 0/SetRumble"() -> (w531:dbl)
    n277 = global read "Robot Global Data.vi" "RollerSolenoidValue"() -> (w517:bool)
    n278 = global read "Robot Global Data.vi" "ElevatorMotorValue"() -> (w584:dbl)
    n279 = Less Or Equal To 0?(x=w503) -> (x <= 0?=w515:bool)
    n280 = global write "Robot Global Data.vi" "EncoderRight"(w509) -> ()
    n281 = global write "Robot Global Data.vi" "EncoderLeft"(w507) -> ()
    n282 = call "TON ONS.vi"("Delay (ms)"=w552, "Input"=w551) -> ("Output 2"=w559:bool)  [unwired: 9 in]
    n283 = call "TON ONS.vi"("Delay (ms)"=w552, "Input"=w550) -> ("Output 2"=w558:bool)  [unwired: 9 in]
    n284 = Decrement(x=w473) -> (x-1=w555:u8)
    n285 = global write "Robot Global Data.vi" "GyroAngle"(w521) -> ()
    n286 = global read "Robot Global Data.vi" "Robot Mode"() -> (w483:T25)
    n287 = Select(t=WPI_SolenoidValue."Forward" ("Value"), s=w541, f=WPI_SolenoidValue."Reverse") -> (s? t:f=w542:T29)
    n288 = Less Or Equal To 0?(x=w511) -> (x <= 0?=w513:bool)
    n289 = call-poly <vilib>:"SD Write Value.vi"("Numeric"=w557, "Name"="AutoToRun") -> ()  [unwired: 8 in, 2 out]
    n290 = call-poly <vilib>:"SD Write Value.vi"("Numeric"=w507, "Name"="EncoderLeft") -> ()  [unwired: 8 in, 2 out]
    n291 = call-poly <vilib>:"SD Write Value.vi"("Numeric"=w509, "Name"="EncoderRight") -> ()  [unwired: 8 in, 2 out]
    n292 = call-poly <vilib>:"WPI_SolenoidSet.vi"("Value"=w542, "SolenoidDevRef"=w544) -> ()  [unwired: 8 in, 2 out]
    n293 = call <vilib>:"WPI_MotorControlSetOutput.vi"("Output"=w505, "MotorControlDevRef"=w528) -> ()  [unwired: 7 in, 3 out]
    n294 = call <vilib>:"WPI_MotorControlSetOutput.vi"("Output"=w505, "MotorControlDevRef"=w527) -> ()  [unwired: 7 in, 3 out]
    n295 = call <vilib>:"WPI_MotorControlSetOutput.vi"("Output"=w587, "MotorControlDevRef"=w588) -> ()  [unwired: 7 in, 3 out]
    n296 = call-poly <vilib>:"WPI_SolenoidSet.vi"("Value"=w543, "SolenoidDevRef"=w573) -> ()  [unwired: 8 in, 2 out]
    n297 = call <vilib>:"WPI_RobotDriveMotors.vi"("RightSpeed"=w585, "LeftSpeed"=w586, "RobotDriveDevRef"=w589) -> ()  [unwired: 6 in, 3 out]
    n298 = And(x=w513, y=w515) -> ()  [unwired: 1 out]
    n299 = Equal?(x=w473, y=9.0) -> (x = y?=w471:bool)
    n300 = Equal?(x=w473, y=10.0) -> (x = y?=w472:bool)
    n301 = Select(t=w555, s=w558, f=w473) -> (s? t:f=w554:u8)
    n302 = Equal?(x=WPI_DriverStationRobotMode2."Teleop Enabled" ("y"), y=w539) -> (x = y?=w533:bool)
    n303 = Equal?(x=WPI_DriverStationRobotMode2."Autonomous Enabled" ("y"), y=w483) -> (x = y?=w482:bool)
    n304 = call-poly <vilib>:"SD Write Value.vi"("Numeric"=w521, "Name"="Gyro0") -> ()  [unwired: 8 in, 2 out]
    n305 = global read "Robot Global Data.vi" "UpperGripperSolenoid"() -> (w499:bool)
    n306 = global read "Robot Global Data.vi" "CanBurglarSolenoidDriver"() -> (w494:bool)
    n307 = call <vilib>:"WPI_MotorControlSetOutput.vi"("Output"=w584, "MotorControlDevRef"=w583) -> ()  [unwired: 7 in, 3 out]
    n308 = global read "Robot Global Data.vi" "DriverResetEncoders"() -> (w493:bool)
    n309 = Select(t=WPI_SolenoidValue."Forward" ("Value"), s=w517, f=WPI_SolenoidValue."Reverse") -> (s? t:f=w524:T29)
    n310 = Equal?(x=WPI_DriverStationRobotMode2."Teleop Disabled" ("y"), y=w483) -> (x = y?=w566:bool)
    n311 = Equal?(x=w483, y=WPI_DriverStationRobotMode2."Autonomous Disabled") -> (x = y?=w565:bool)
    n312 = Increment(x=w554) -> (x+1=w553:u8)
    n313 = Select(t=w531, s=w533, f=0.0) -> (s? t:f=w532:dbl)
    n314 = call "TOF ONS.vi"("Delay (ms)"=u32 500, "Input"=w482) -> ("Output"=w481:bool)  [unwired: 9 in]
    n315 = call-poly <vilib>:"WPI_SolenoidSet.vi"("Value"=w524, "SolenoidDevRef"=w526) -> ()  [unwired: 8 in, 2 out]
    n316 = call <vilib>:"WPI_JoystickSetOutputs.vi"("Right Rumble"=w532, "Left Rumble"=w532, "JoystickDevRef"=w530) -> ()  [unwired: 7 in, 2 out]
    n317 = Select(t=w553, s=w559, f=w554) -> (s? t:f=w560:u8)
    n318 = Or(x=w566, y=w565) -> (x .or. y?=w568:bool)
    n319 = Not(x=w570) -> (.not. x?=w506:bool)
    "GoatDetectorPhotoeye" <- w506
    n320 = Select(t=0.0, s=FALSE, f=w511) -> (s? t:f=w512:dbl)
    n321 = call "TOF.vi"("Delay (ms)"=u32 500, "Input"=w481) -> ("Output"=w478:bool)  [unwired: 9 in]
    n322 = call <vilib>:"WPI_MotorControlSetOutput.vi"("Output"=w512, "MotorControlDevRef"=w518) -> ()  [unwired: 7 in, 3 out]
    n323 = global write "Robot Global Data.vi" "GoatDetectorPhotoeye"(w506) -> ()
    n324 = case shown="True" w493 {
      tunnel: w492 -> [_ w590]
      tunnel: w491 -> [_ w591]
      frame False {
      }
      frame True {
        n325 = call <vilib>:"WPI_EncoderReset.vi"("EncoderDevRef"=w590) -> ()  [unwired: 9 in, 2 out]
        n326 = call <vilib>:"WPI_EncoderReset.vi"("EncoderDevRef"=w591) -> ()  [unwired: 9 in, 2 out]
      }
    }
    n327 = Select(t=WPI_SolenoidValue."On" ("Value"), s=w499, f=WPI_SolenoidValue."Off") -> (s? t:f=w498:T29)
    n328 = call-poly <vilib>:"WPI_SolenoidSet.vi"("Value"=w498, "SolenoidDevRef"=w502) -> ()  [unwired: 8 in, 2 out]
    n329 = Select(t=w488, s=w533, f=0.0) -> (s? t:f=w535:dbl)
    n330 = In Range and Coerce(upper limit=u8 11, x=w560, lower limit=u8 0) -> (coerced(x)=w490:u8)  [unwired: 1 out]
    n331 = Or(x=w471, y=w472) -> (x .or. y?=w479:bool)
    n332 = Select(t=w490, s=w568, f=w473) -> (s? t:f=w567:u8)
    n333 = call <vilib>:"WPI_JoystickSetOutputs.vi"("Right Rumble"=w535, "Left Rumble"=w535, "JoystickDevRef"=w537) -> ()  [unwired: 7 in, 2 out]
    n334 = And(x=w478, y=w479) -> (x .and. y?=w480:bool)
    n335 = Or(x=w480, y=w494) -> (x .or. y?=w485:bool)
    n336 = global write "Auto_Conf.vi" "AutoToRun"(w567) -> ()
    n337 = Wait Until Next ms Multiple(millisecond multiple=u32 20 ("milliseconds to wait")) -> ()  [unwired: 1 out]
    n338 = Select(t=WPI_SolenoidValue."On" ("Value"), s=w485, f=WPI_SolenoidValue."Off") -> (s? t:f=w487:T29)
    n339 = call-poly <vilib>:"WPI_SolenoidSet.vi"("Value"=w487, "SolenoidDevRef"=w497) -> ()  [unwired: 8 in, 2 out]
    n340 = call-poly <vilib>:"WPI_SolenoidSet.vi"("Value"=w487, "SolenoidDevRef"=w486) -> ()  [unwired: 8 in, 2 out]
  }
  n341 = while {
    stop <- FALSE stop-if-true
    # "Power Distribution Panel - Get Voltage"
    # "Power Distribution Panel - Get Current"
    n342 = call <vilib>:"WPI_Power Get PCM Compressor Current.vi"() -> ("current (A)"=w593:dbl)  [unwired: 14 in, 1 out]
    n343 = call <vilib>:"WPI_Power Get PDP Voltage.vi"("Power Distribution Panel (0)"=u8 0) -> ("voltage (V)"=w594:dbl)  [unwired: 13 in, 1 out]
    "Voltage" <- w594
    n344 = Wait (ms)(milliseconds to wait=u32 50) -> ()  [unwired: 1 out]
    n345 = global write "Robot Global Data.vi" "CompressorAmperage"(w593) -> ()
    n346 = call <vilib>:"WPI_Power Get PDP Currents.vi"("Power Distribution Panel (0)"=u8 0, "PDP Channel"=13) -> ("current (A)"=w595:dbl, "all currents (A)"=w600:dbl[])  [unwired: 11 in, 1 out]
    "ElevatorCurrent" <- w595
    n347 = Add Array Elements(numeric array=w600) -> (sum=→"CurrentSum":dbl)
    n348 = global write "Robot Global Data.vi" "ElevatorAmperage"(w595) -> ()
    n349 = global write "Robot Global Data.vi" "BatteryVoltage"(w594) -> ()
  }
